vi "ROTPENT_Disturbance.vi"(1 "Vi":dbl, 2 "Apply Disturbance":bool) -> (0 "Vm":dbl)   [LabVIEW 2021]
doc: "Adds a disturbance voltage of Vsd to the input motor voltage Vi. The resulting\napplied voltage is Vm = Vi + Vsd."
panel:
  in  "Vsd":dbl=5.0
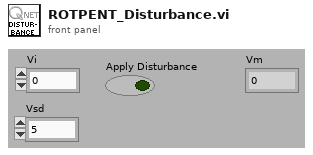
[diagram p1: front panel]
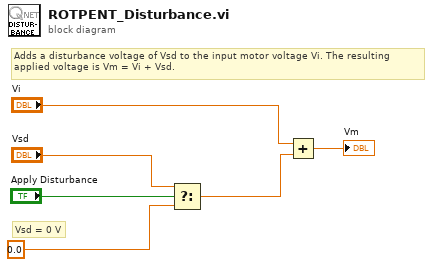
[diagram p0: block diagram]
diagram:
  # "Adds a disturbance voltage of Vsd to the input motor voltage Vi. The resulting\napplied voltage is Vm = Vi + Vsd."
  # "Vsd = 0 V"
  n1 = Select(t="Vsd", s="Apply Disturbance", f=0.0) -> (s? t:f=w2:dbl)
  n2 = Add(x="Vi", y=w2) -> (x+y=→"Vm":dbl)
